vi "Read Current Setpoint (Single).vi"(8 "error in":errorcluster, 9 "Channel Index":i32=1, 11 "Current Control in":refnum<class "Current Control.lvclass">) -> (0 "error out":errorcluster, 1 "Changed or First Call?":bool, 2 "Current Setpoint":dbl, 3 "Current Control out":refnum<class "Current Control.lvclass">)   [LabVIEW 2023, in "Current Control.lvclass"]
doc: "This VI will read a single Channel's setpoint. The <b>Channel Index</b> input is 1-based."
uses:
  Current Control.lvclass
  Current Control.lvclass/Current Control.ctl
  <vilib>/ADAS Replay HIL/Channels/Tag Wrapper/Polymorphic/Read Channel (Double).vi
  49ccd0c4-676c-49c2-8dbb-76c3f60c238e.vi
  <vilib>/ADAS Replay HIL/Channels/Tag Wrapper/Polymorphic/Read Channel (Double).vi/b2f764de-0c1e-4784-a155-687fc995a684.vi
  <vilib>/ADAS Replay HIL/Channels/Tag Wrapper/Polymorphic/Read Channel (Double).vi/b2f764de-0c1e-4784-a155-687fc995a684.vi/c28b0ead-42ad-4072-80a2-aca7f2bd7ce3.vi
  <vilib>/ADAS Replay HIL/Channels/Tag Wrapper/Polymorphic/Read Channel (Double).vi/b2f764de-0c1e-4784-a155-687fc995a684.vi/219d0231-d98b-4193-b5cc-84f90e3c9091.vi
  <vilib>/ADAS Replay HIL/Channels/Tag Wrapper/Tag Wrapper.lvlib
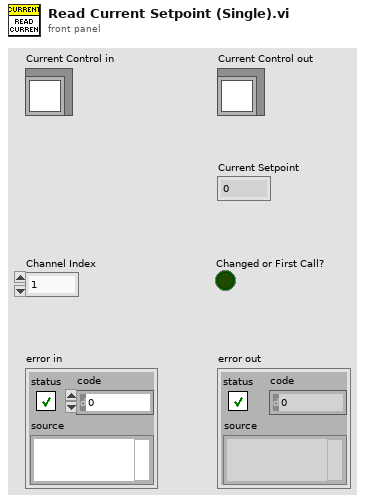
[diagram p1: front panel]
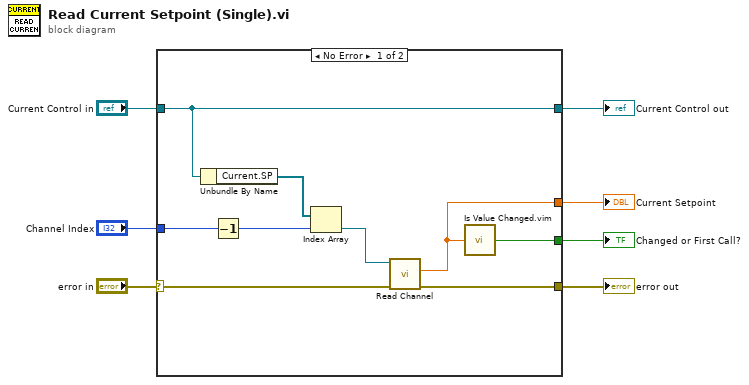
[diagram p0: block diagram]
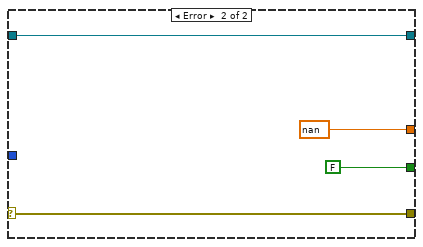
[diagram p2: hidden frame]
diagram:
  n1 = case shown="No Error" "error in" {
    selector: "error in" -> [w14 w20]
    tunnel: [w13 w20] -> w6
    tunnel: [w16 w19] -> w4
    tunnel: "Current Control in" -> [w16 w19]
    tunnel: [w12 nan] -> w2
    tunnel: [w11 FALSE ("changed or first call?")] -> w3
    tunnel: "Channel Index" -> [w9 _]
    frame No Error {
      n2 = Unbundle By Name(w16) -> ("Current.SP"=w15:refnum<k21>[])
      n3 = Decrement(x=w9) -> (x-1=w8:i32)
      n4 = Index Array(array=w15, index=w8) -> (element=w10:refnum<k21>)
      n5 = call-poly <vilib>:"Read Channel.vi"("error in"=w14, "ADAS HIL Channel in"=w10) -> ("error out"=w13:errorcluster, "Value out"=w12:dbl)  [unwired: 6 in, 2 out]
      n6 = call "Is Value Changed.vim"("value"=w12) -> ("changed or first call?"=w11:bool)
    }
    frame Error {
    }
  }
  "error out" <- w6
  "Current Control out" <- w4
  "Changed or First Call?" <- w3
  "Current Setpoint" <- w2
